vi "Read Type.vi"(8 "Error In":errorcluster, 11 "Pre-Render Variable In":refnum<class "Variable.lvclass">) -> (0 "Error Out":errorcluster, 2 "Type":T1=enum."Render Variable", 3 "Pre-Render Variable Out":refnum<class "Variable.lvclass">)   [LabVIEW 2018, in "Toolkit.lvlib" / "Hooks.lvlib" / "Render.lvlib" / "Variable.lvclass"]
uses:
  Variable.lvclass
  Type Definitions/Types.ctl
  Hooks.lvlib
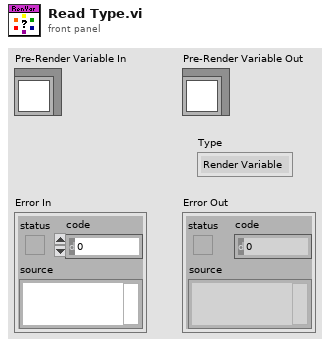
[diagram p1: front panel]
types:
  T1 = typedef "Toolkit.lvlib/Hooks.lvlib/Types.ctl" = enum16{"Unknown", "Render Variable", "Render Section"}
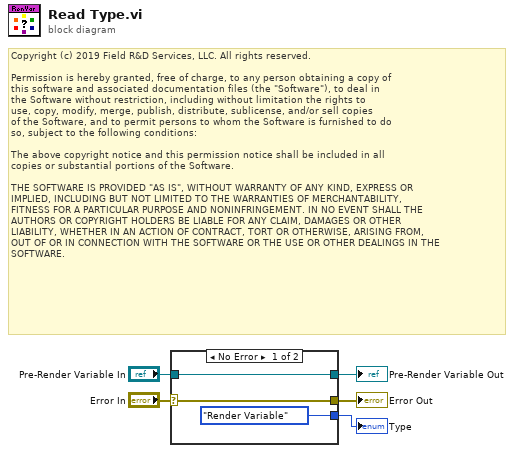
[diagram p0: block diagram]
diagram:
  # "Copyright (c) 2019 Field R&D Services, LLC. All rights reserved.\n\nPermission is hereby granted, free of charge, to any person obtaining a copy of\nthis software and associated documentation files (the \"Software\"), to deal in\nthe Software without restriction, including without limitation the rights to\nuse, copy, modify, merge, publish, distribute, sublicense, and/or sell copies\nof the Software, and to permit persons to whom the Software is furnished to do\nso, subject to the following conditions:\n\nThe above copyright notice and this permission notice shall be included in all\ncopies or substantial portions of the Software.\n\nTHE SOFTWARE IS PROVIDED \"AS IS\", WITHOUT WARRANTY OF ANY KIND, EXPRESS OR\nIMPLIED, INCLUDING BUT NOT LIMITED TO THE WARRANTIES OF MERCHANTABILITY,\nFITNESS FOR A PARTICULAR PURPOSE AND NONINFRINGEMENT. IN NO EVENT SHALL THE\nAUTHORS OR COPYRIGHT HOLDERS BE LIABLE FOR ANY CLAIM, DAMAGES OR OTHER\nLIABILITY, WHETHER IN AN ACTION OF CONTRACT, TORT OR OTHERWISE, ARISING FROM,\nOUT OF OR IN CONNECTION WITH THE SOFTWARE OR THE USE OR OTHER DEALINGS IN THE\nSOFTWARE."
  n1 = case shown="No Error" "Error In" {
    selector: "Error In" -> [w7 w9]
    tunnel: [w8 w10] -> w4
    tunnel: "Pre-Render Variable In" -> [w8 w10]
    tunnel: [w7 w9] -> w2
    tunnel: [Types."Render Variable" ("Type") _] -> w1
    frame No Error {
    }
    frame Error {
    }
  }
  "Error Out" <- w2
  "Pre-Render Variable Out" <- w4
  "Type" <- w1
